vi "chenillard.vi"() -> ()   [LabVIEW 2025]
panel:
  out "d3":bool
  out "d2":bool
  out "d1":bool
  out "d0":bool
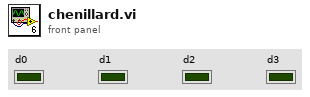
[diagram p1: front panel]
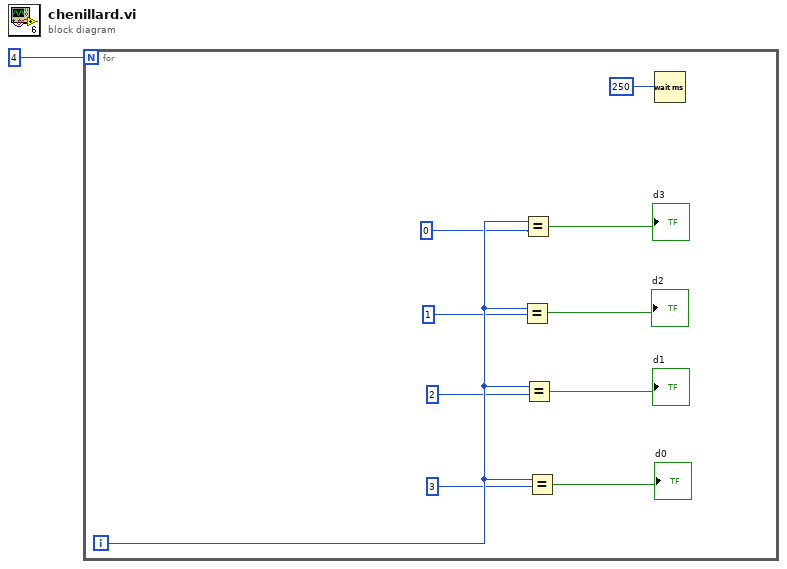
[diagram p0: block diagram]
diagram:
  n1 = for {
    N: 4 -> [_]
    i -> [w10]
    n2 = Equal?(x=w10, y=1) -> (x = y?=→"d2":bool)
    n3 = Equal?(x=w10, y=0) -> (x = y?=→"d3":bool)
    n4 = Equal?(x=w10, y=2) -> (x = y?=→"d1":bool)
    n5 = Equal?(x=w10, y=3) -> (x = y?=→"d0":bool)
    n6 = Wait (ms)(milliseconds to wait=250) -> ()  [unwired: 1 out]
  }
